vi "p2.vi"() -> ()   [LabVIEW 2021, in "d17.lvlib"]
uses:
  d17.lvlib
  8c3191a2-c781-462e-8e95-00f0ede287dc.vi
  <vilib>/Comparison/Less/Less Functor/Less Functor.lvclass
  AOC/AOC.lvlib
panel:
  out "Shapes Array":i32[](array[numeric])
  out "Height Array":i32[](array[numeric])
  out "Answer":u64
  out "height":i32
  out "Delta height":i32
  out "Heght at 1st repeat":i32
  out "Heght at 2nd repeat":i32
  out "Delta shapes":i32
  out "Shapes at 2nd repeat":i32
  out "Shapes at 1st repeat":i32
  in  "max shapes":u64=2022
  out "shape count":u64=2022
  out "XY Graph":cluster{cluster{"x":i32, "y":i32}[]}[](graph)
  in  "Example":string=">>><<><>><<<>><>>><<<>>><<<><<<>><>><<>>"
  in  "Example":bool
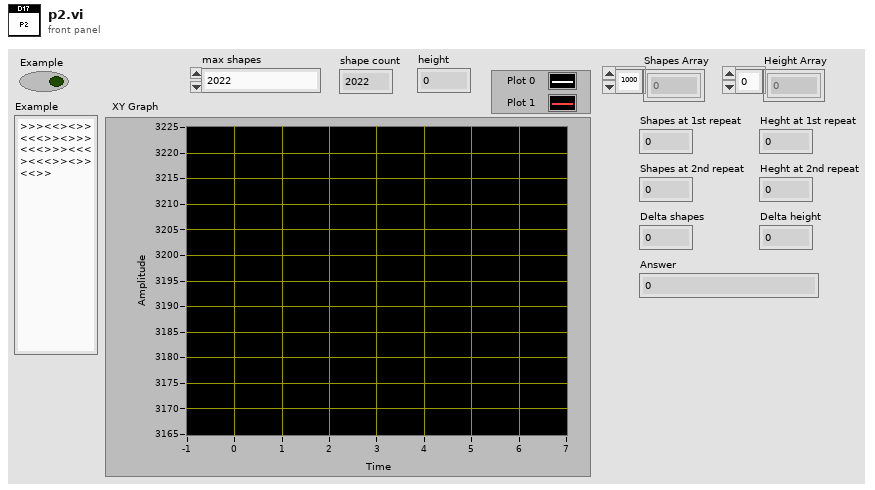
[diagram p1: front panel]
types:
  T1 = cluster{"Co-ordinates":cluster{"x":i8, "y":i8}[]}
  T2 = cluster{"Co-ordinates":cluster{"x":i8, "y":i8}[]}[]
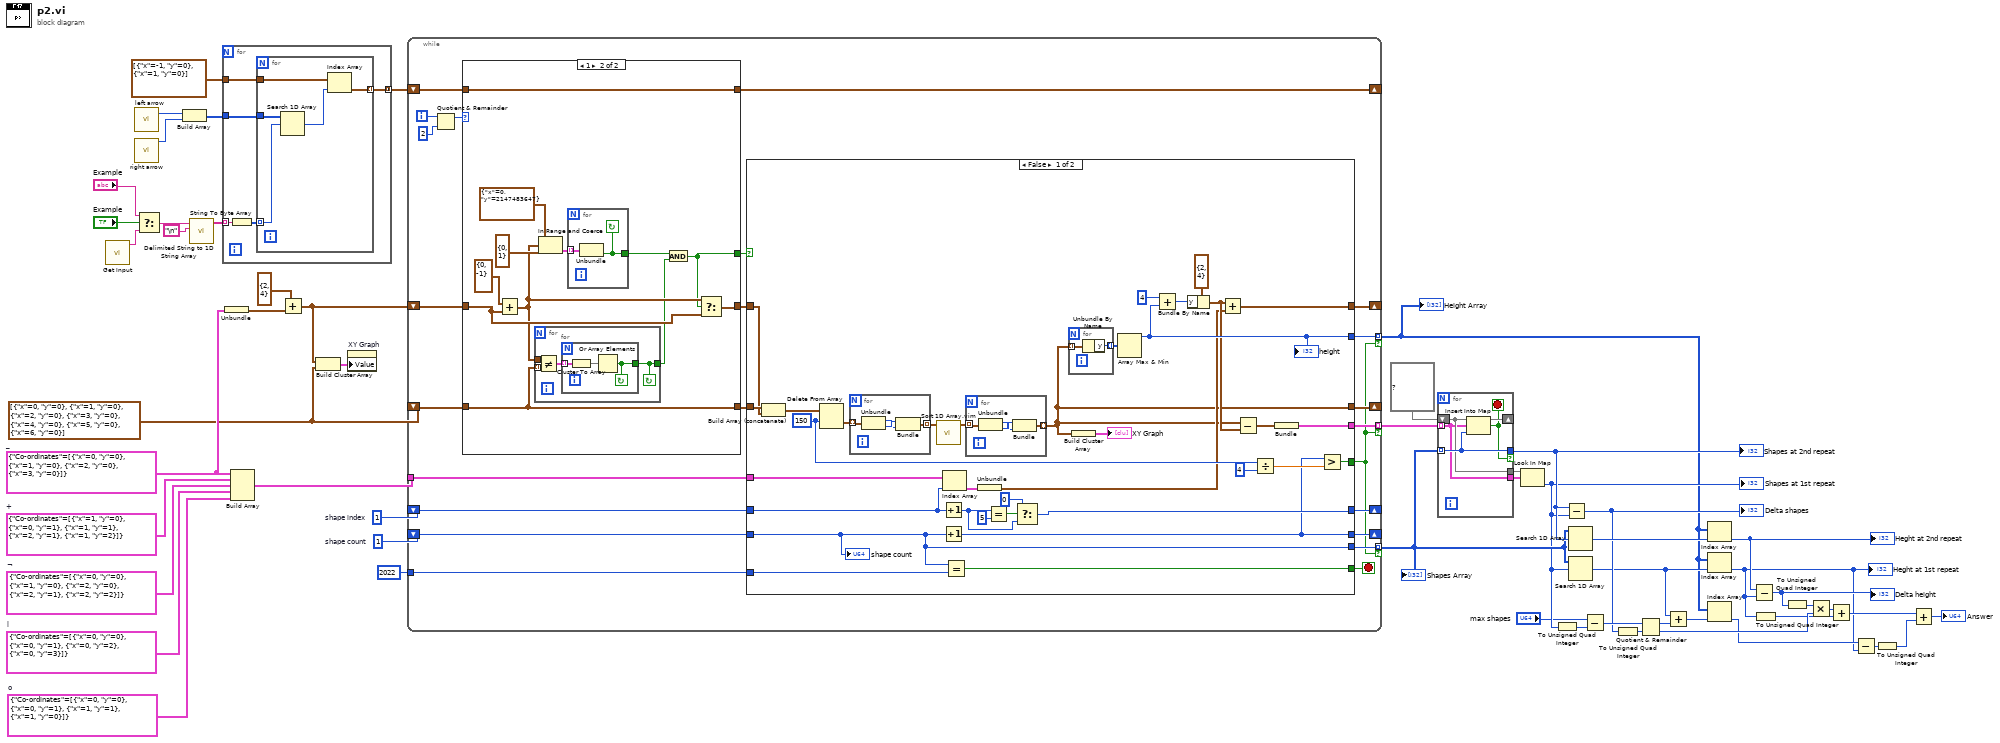
[diagram p0: block diagram]
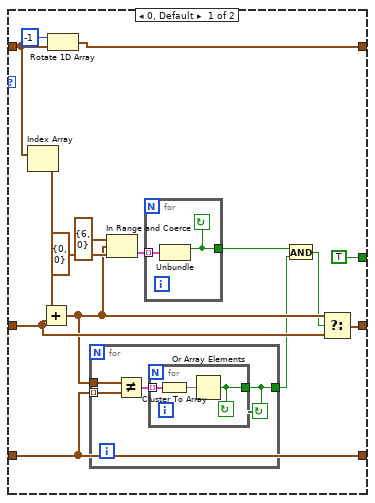
[diagram p3: hidden frame]
diagram:
  w32 = cluster{"x":i32, "y":i32}[] [{"x"=0, "y"=0}, {"x"=1, "y"=0}, {"x"=2, "y"=0}, {"x"=3, "y"=0}, {"x"=4, "y"=0}, {"x"=5, "y"=0}, {"x"=6, "y"=0}]
  w37 = 1  # shape count
  w38 = 1  # shape index
  w40 = T1 {"Co-ordinates"=[{"x"=0, "y"=0}, {"x"=0, "y"=1}, {"x"=1, "y"=1}, {"x"=1, "y"=0}]}  # o
  w41 = T1 {"Co-ordinates"=[{"x"=0, "y"=0}, {"x"=0, "y"=1}, {"x"=0, "y"=2}, {"x"=0, "y"=3}]}  # l
  w42 = T1 {"Co-ordinates"=[{"x"=0, "y"=0}, {"x"=1, "y"=0}, {"x"=2, "y"=0}, {"x"=2, "y"=1}, {"x"=2, "y"=2}]}  # ¬
  w43 = T1 {"Co-ordinates"=[{"x"=1, "y"=0}, {"x"=0, "y"=1}, {"x"=1, "y"=1}, {"x"=2, "y"=1}, {"x"=1, "y"=2}]}  # +
  w36 = T1 {"Co-ordinates"=[{"x"=0, "y"=0}, {"x"=1, "y"=0}, {"x"=2, "y"=0}, {"x"=3, "y"=0}]}  # _
  n1 = call "Get Input.vi"() -> ("Input"=w54:string)  [unwired: 11 in]
  n2 = call "left arrow.vi"() -> ("<"=w47:u8)  [unwired: 11 in]
  n3 = call "right arrow.vi"() -> (">"=w46:u8)  [unwired: 11 in]
  n4 = Select(t="Example", s="Example", f=w54) -> (s? t:f=w53:string)
  n5 = Build Array(w47, w46) -> (w45:u8[])
  n6 = call <vilib>:"Delimited String to 1D String Array.vi"("delimiter"="\n", "delimited string"=w53) -> ("string array"=w49:string[])  [unwired: 9 in]
  n7 = for {
    tunnel: w49 -> [w59] mode=indexing
    tunnel: cluster{"x":i8, "y":i8}[] [{"x"=-1, "y"=0}, {"x"=1, "y"=0}] -> [w56]
    tunnel: w45 -> [w57]
    tunnel: [w55] -> w44 mode=concatenating
    n8 = String To Byte Array(string=w59) -> (unsigned byte array=w58:u8[])
    n9 = for {
      tunnel: w58 -> [w63] mode=indexing
      tunnel: w57 -> [w64]
      tunnel: w56 -> [w62]
      tunnel: [w60] -> w55 mode=indexing
      n10 = Search 1D Array(1D array=w64, element=w63) -> (index of element=w61:i32)  [unwired: 1 in]
      n11 = Index Array(array=w62, index=w61) -> (element=w60:cluster{"x":i8, "y":i8})
    }
  }
  n12 = Unbundle(w36) -> ("Co-ordinates"=w35:cluster{"x":i8, "y":i8}[])
  n13 = Build Array(w36, w43, w42, w41, w40) -> (w39:T2)
  n14 = Add(x=cluster{"x":i8, "y":i8} {"x"=2, "y"=4}, y=w35) -> (x+y=w33:cluster{"x":i8, "y":i8}[])
  n15 = Build Cluster Array(w33, w32) -> (w31:cluster{cluster{"x":i32, "y":i32}[]}[])
  n16 = property on="XY Graph" class="XYGraph (strict)"("Value"=w31) -> ()  [unwired: 2 in, 2 out]
  n17 = while {
    shift-right: [w79] -> _
    shift-left: w44 -> [w87]
    tunnel: w39 -> [w86]
    shift-right: [w84] -> _
    shift-left: w38 -> [w85]
    shift-right: [w72] -> _
    shift-left: w33 -> [w78]
    shift-right: [w68] -> _
    shift-left: w37 -> [w70]
    shift-right: [w69] -> _
    shift-left: w32 -> [w75]
    tunnel: [w73] -> w1 mode=indexing if=w65
    tunnel: u64 2022 ("max shapes") -> [w71]
    tunnel: [w67] -> w30 mode=indexing if=w65
    tunnel: [w66] -> w25 mode=indexing if=w65
    i -> [w81]
    stop <- w83 stop-if-true
    n18 = Quotient & Remainder(x=w81, y=2) -> (x-y*floor(x/y)=w82:i32)  [unwired: 1 out]
    n19 = case shown="1" w82 {
      tunnel: w87 -> [w143 w171]
      tunnel: [w149 w171] -> w79
      tunnel: w78 -> [w145 w167]
      tunnel: [w146 w168] -> w77
      tunnel: [TRUE ("y") w162] -> w76
      tunnel: w75 -> [w140 w163]
      tunnel: [w140 w163] -> w74
      frame 0, Default {
        n20 = Index Array(array=w143) -> (element=w138:cluster{"x":i8, "y":i8})  [unwired: 1 in]
        n21 = Add(x=w138, y=w145) -> (x+y=w141:cluster{"x":i32, "y":i32}[])
        n22 = Rotate 1D Array(1:w143, 2:-1 ("n")) -> (0:w149:cluster{"x":i8, "y":i8}[])
        n23 = for {
          tunnel: w141 -> [w152]
          tunnel: w140 -> [w151] mode=indexing
          tunnel: [w154] -> w137
          stop <- w154 continue-if-true
          n24 = Not Equal?(x=w152, y=w151) -> (x != y?=w153:cluster{"x":bool, "y":bool}[])
          n25 = for {
            tunnel: w153 -> [w157] mode=indexing
            tunnel: [w155] -> w154
            stop <- w155 continue-if-true
            n26 = Cluster To Array(cluster=w157) -> (array=w156:bool[])
            n27 = Or Array Elements(Boolean array=w156) -> (logical OR=w155:bool)
          }
        }
        n28 = In Range and Coerce(upper limit=cluster{"x":i8, "y":i8} {"x"=6, "y"=0} ("lower limit"), x=w141, lower limit=cluster{"x":i8, "y":i8} {"x"=0, "y"=0}) -> (In Range?=w136:cluster{"x":bool, "y":bool}[])  [unwired: 1 out]
        n29 = for {
          tunnel: w136 -> [w159] mode=indexing
          tunnel: [w158] -> w144
          stop <- w158 continue-if-true
          n30 = Unbundle(w159) -> ("x"=w158:bool)  [unwired: 1 out]
        }
        n31 = And(x=w144, y=w137) -> (x .and. y?=w139:bool)
        n32 = Select(t=w141, s=w139, f=w145) -> (s? t:f=w146:cluster{"x":i32, "y":i32}[])
      }
      frame 1 {
        n33 = Add(x=cluster{"x":i8, "y":i8} {"x"=0, "y"=-1}, y=w167) -> (x+y=w164:cluster{"x":i32, "y":i32}[])
        n34 = for {
          tunnel: w164 -> [w175]
          tunnel: w163 -> [w174] mode=indexing
          tunnel: [w172] -> w161
          stop <- w172 continue-if-true
          n35 = Not Equal?(x=w175, y=w174) -> (x != y?=w173:cluster{"x":bool, "y":bool}[])
          n36 = for {
            tunnel: w173 -> [w178] mode=indexing
            tunnel: [w176] -> w172
            stop <- w176 continue-if-true
            n37 = Cluster To Array(cluster=w178) -> (array=w177:bool[])
            n38 = Or Array Elements(Boolean array=w177) -> (logical OR=w176:bool)
          }
        }
        n39 = In Range and Coerce(upper limit=cluster{"x":i32, "y":i32} {"x"=0, "y"=2147483647}, x=w164, lower limit=cluster{"x":i8, "y":i8} {"x"=0, "y"=1}) -> (In Range?=w169:cluster{"x":bool, "y":bool}[])  [unwired: 1 out]
        n40 = for {
          tunnel: w169 -> [w180] mode=indexing
          tunnel: [w179] -> w166
          stop <- w179 continue-if-true
          n41 = Unbundle(w180) -> ("y"=w179:bool)  [unwired: 1 out]
        }
        n42 = And(x=w166, y=w161) -> (x .and. y?=w162:bool)
        n43 = Select(t=w164, s=w162, f=w167) -> (s? t:f=w168:cluster{"x":i32, "y":i32}[])
      }
    }
    n44 = case shown="False" w76 {
      tunnel: w86 -> [w121 _]
      tunnel: w85 -> [w119 w135]
      tunnel: [w113 w135] -> w84
      tunnel: [w116 w133] -> w72
      tunnel: w77 -> [w106 w133]
      tunnel: w70 -> [w89 w134]
      tunnel: [w93 w134] -> w68
      tunnel: [w110 _] -> w83
      tunnel: [w88 w132] -> w69
      tunnel: w74 -> [w109 w132]
      tunnel: [w104 _] -> w73
      tunnel: w71 -> [w105 _]
      tunnel: [w91 _] -> w67
      tunnel: [w94 _] -> w65
      tunnel: [w89 _] -> w66
      frame False {
        w97 = 150 ("length")
        n45 = Build Array (concatenate)(w109, w106) -> (w103:cluster{"x":i32, "y":i32}[])
        n46 = Delete From Array(array=w103, length=w97) -> (deleted portion=w102:cluster{"x":i32, "y":i32}[])  [unwired: 1 in, 1 out]
        n47 = for {
          tunnel: w102 -> [w129] mode=indexing
          tunnel: [w126] -> w101 mode=indexing
          n48 = Unbundle(w129) -> ("x"=w127:i32, "y"=w128:i32)
          n49 = Bundle("y"=w128, "x"=w127) -> (w126:cluster{"y":i32, "x":i32})  [unwired: 1 in]
        }
        n50 = call "Sort 1D Array.vim"("unsorted array"=w101) -> ("sorted array"=w100:cluster{"y":i32, "x":i32}[])  [unwired: 10 in]
        n51 = Increment(x=w119) -> (x+1=w112:i32)
        n52 = Increment(x=w89) -> (x+1=w93:i32)
        n53 = Index Array(array=w121, index=w119) -> (element=w120:T1)
        n54 = Equal?(x=w89, y=w105) -> (x = y?=w110:bool)
        n55 = for {
          tunnel: w100 -> [w125] mode=indexing
          tunnel: [w122] -> w88 mode=indexing
          n56 = Unbundle(w125) -> ("y"=w123:i32, "x"=w124:i32)
          n57 = Bundle("x"=w124, "y"=w123) -> (w122:cluster{"x":i32, "y":i32})  [unwired: 1 in]
        }
        n58 = Unbundle(w120) -> ("Co-ordinates"=w90:cluster{"x":i8, "y":i8}[])
        n59 = Equal?(x=w112, y=5) -> (x = y?=w114:bool)
        n60 = Select(t=0, s=w114, f=w112) -> (s? t:f=w113:i32)
        n61 = for {
          tunnel: w88 -> [w131] mode=indexing
          tunnel: [w130] -> w108 mode=indexing
          n62 = Unbundle By Name(w131) -> ("y"=w130:i32)
        }
        n63 = Build Cluster Array(w88) -> (→"XY Graph":cluster{cluster{"x":i32, "y":i32}[]}[])
        n64 = Array Max & Min(array=w108) -> (max value=w104:i32)  [unwired: 3 out]
        "height" <- w104
        n65 = Add(x=4, y=w104) -> (x+y=w117:i32)
        n66 = Bundle By Name(cluster=cluster{"x":i32, "y":i32} {"x"=2, "y"=4} ("Co-ordinate"), "y"=w117) -> (w99:cluster{"x":i32, "y":i32})
        n67 = Add(x=w99, y=w90) -> (x+y=w116:cluster{"x":i32, "y":i32}[])
        n68 = Subtract(x=w88, y=w99) -> (x-y=w92:cluster{"x":i32, "y":i32}[])
        n69 = Divide(x=w97, y=4) -> (x/y=w96:dbl)
        n70 = Bundle(w92) -> (w91:cluster{cluster{"x":i32, "y":i32}[]})  [unwired: 1 in]
        n71 = Greater?(x=w93, y=w96) -> (0:w94:bool)
        "shape count" <- w89
      }
      frame True {
      }
    }
  }
  "Height Array" <- w1
  "Shapes Array" <- w25
  n72 = for {
    tunnel: w30 -> [w181] mode=indexing
    tunnel: w25 -> [w184] mode=indexing
    shift-right: [w185] -> _
    shift-left: map{cluster{cluster{"x":i32, "y":i32}[]}, i32} {} ("map in") -> [w182]
    tunnel: [w184] -> w26 if=w183
    tunnel: [w182] -> w28
    tunnel: [w181] -> w27
    stop <- w183 stop-if-true
    n73 = Insert Into Map(map in=w182, key=w181, value=w184) -> (map out=w185:map{cluster{cluster{"x":i32, "y":i32}[]}, i32}, key already included?=w183:bool)  [unwired: 1 out]
  }
  "Shapes at 2nd repeat" <- w26
  n74 = Look In Map(map=w28, key=w27) -> (value=w22:i32)  [unwired: 1 in, 1 out]
  "Shapes at 1st repeat" <- w22
  n75 = To Unsigned Quad Integer(1:w22) -> (0:w3:u64)
  n76 = Subtract(x=w26, y=w22) -> (x-y=w19:i32)
  "Delta shapes" <- w19
  n77 = Search 1D Array(1D array=w25, element=w26) -> (index of element=w24:i32)  [unwired: 1 in]
  n78 = Search 1D Array(1D array=w25, element=w22) -> (index of element=w11:i32)  [unwired: 1 in]
  n79 = Subtract(x="max shapes", y=w3) -> (x-y=w20:u64)
  n80 = To Unsigned Quad Integer(1:w19) -> (0:w2:u64)
  n81 = Quotient & Remainder(x=w20, y=w2) -> (x-y*floor(x/y)=w12:u64, floor(x/y)=w18:u64)
  n82 = Add(x=w11, y=w12) -> (x+y=w10:u64)
  n83 = Index Array(array=w1, index=w24) -> (element=w23:i32)
  "Heght at 2nd repeat" <- w23
  n84 = Index Array(array=w1, index=w11) -> (element=w8:i32)
  "Heght at 1st repeat" <- w8
  n85 = Index Array(array=w1, index=w10) -> (element=w9:i32)
  n86 = Subtract(x=w23, y=w8) -> (x-y=w17:i32)
  "Delta height" <- w17
  n87 = To Unsigned Quad Integer(1:w8) -> (0:w14:u64)
  n88 = To Unsigned Quad Integer(1:w17) -> (0:w15:u64)
  n89 = Multiply(x=w15, y=w18) -> (x*y=w16:u64)
  n90 = Add(x=w16, y=w14) -> (x+y=w13:u64)
  n91 = Subtract(x=w9, y=w8) -> (x-y=w6:i32)
  n92 = To Unsigned Quad Integer(1:w6) -> (0:w5:u64)
  n93 = Add(x=w13, y=w5) -> (x+y=→"Answer":u64)
